vi "Actividad 2.vi"() -> ()   [LabVIEW 2020]
uses:
  <vilib>/httpClient/LabVIEWHTTPClient.lvlib
panel:
  out "Humedad":dbl
  out "Fecha":string
  out "Temperatura":dbl
  out "Lateral":bool
  out "error GET 2":errorcluster
  out "Frontal":bool
  out "body GET":string
  out "headers GET":string
  in  "stop":bool
  out "error GET":errorcluster
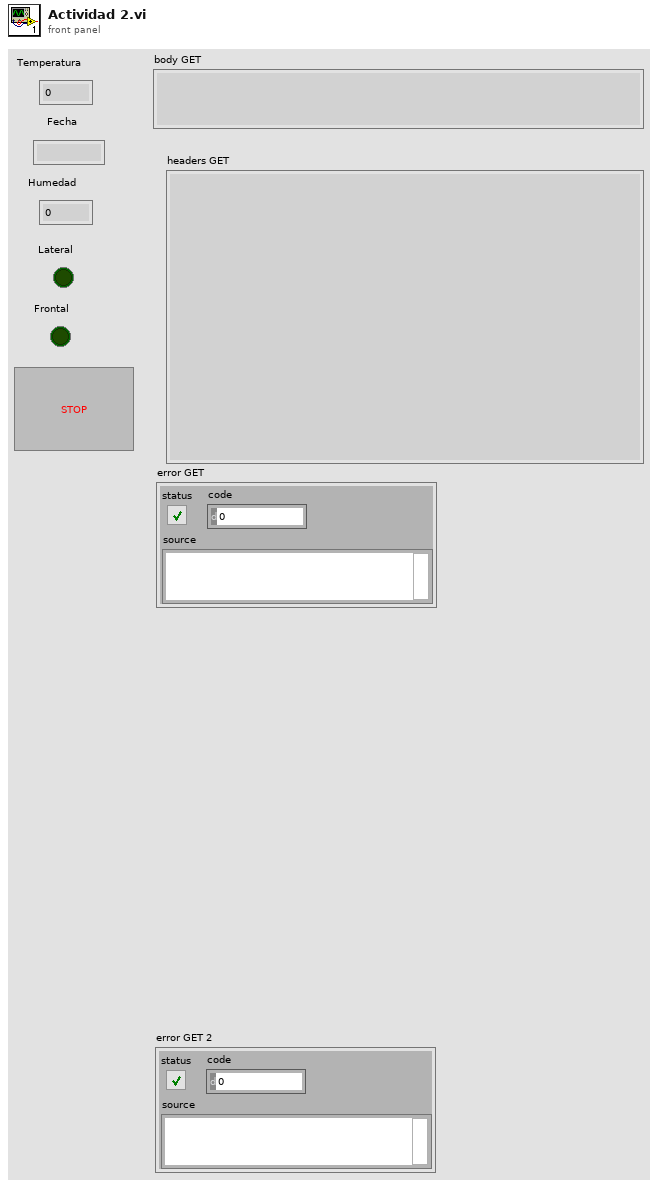
[diagram p1: front panel]
types:
  T1 = cluster{"Temperatura":dbl, "Fecha":string, "Humedad":dbl}
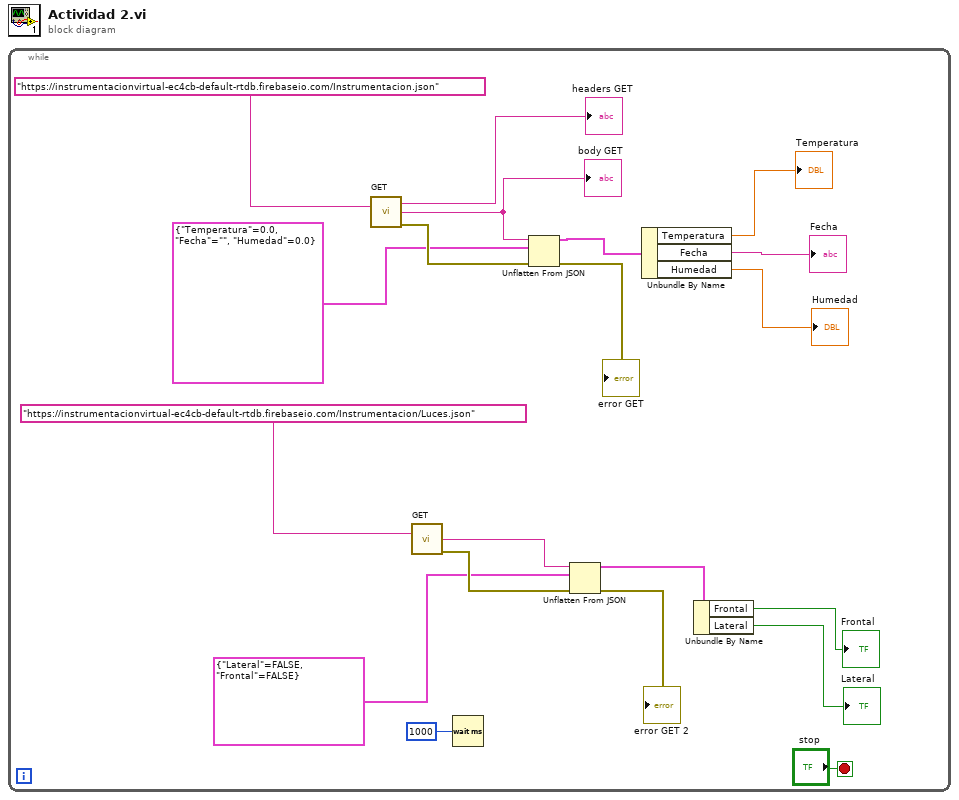
[diagram p0: block diagram]
diagram:
  n1 = while {
    stop <- "stop" stop-if-true
    n2 = call <vilib>:"GET.vi"("url"="https://instrumentacionvirtual-ec4cb-default-rtdb.firebaseio.com/Instrumentacion.json") -> ("headers"=→"headers GET":string, "body"=w15:string, "error out"=w16:errorcluster)  [unwired: 11 in, 1 out]
    "body GET" <- w15
    n3 = call <vilib>:"GET.vi"("url"="https://instrumentacionvirtual-ec4cb-default-rtdb.firebaseio.com/Instrumentacion/Luces.json") -> ("body"=w9:string, "error out"=w10:errorcluster)  [unwired: 11 in, 2 out]
    n4 = Wait (ms)(milliseconds to wait=u32 1000) -> ()  [unwired: 1 out]
    n5 = Unflatten From JSON(JSON string=w15, type and defaults=T1 {"Temperatura"=0.0, "Fecha"="", "Humedad"=0.0}, error in (no error)=w16) -> (value=w4:T1, error out=→"error GET":errorcluster)  [unwired: 4 in]
    n6 = Unflatten From JSON(JSON string=w9, type and defaults=cluster{"Lateral":bool, "Frontal":bool} {"Lateral"=FALSE, "Frontal"=FALSE}, error in (no error)=w10) -> (value=w7:cluster{"Lateral":bool, "Frontal":bool}, error out=→"error GET 2":errorcluster)  [unwired: 4 in]
    n7 = Unbundle By Name(w4) -> ("Temperatura"=→"Temperatura":dbl, "Fecha"=→"Fecha":string, "Humedad"=→"Humedad":dbl)
    n8 = Unbundle By Name(w7) -> ("Frontal"=→"Frontal":bool, "Lateral"=→"Lateral":bool)
  }
